vi "test_next_steps_json.vi"(8 "error in (no error)":errorcluster) -> (0 "error out":errorcluster)   [LabVIEW 2023, in "Easy.SequenceManager.Test.lvlib"]
uses:
  Easy.SequenceManager.Test.lvlib
  src/SequenceManager/SequenceManager.lvclass
  <vilib>/addons/_JKI Toolkits/Caraya/classes/Assert/Assert Equal Value and Type_Variant.vi
  <vilib>/addons/_JKI Toolkits/Caraya/classes/Test/Test.lvclass
  <vilib>/addons/_JKI Toolkits/Caraya/classes/Assert/Assert.lvclass
panel:
  in  "SequenceManager in":refnum<class "SequenceManager.lvclass">
  # "Connector Pane"
  # "Locals"
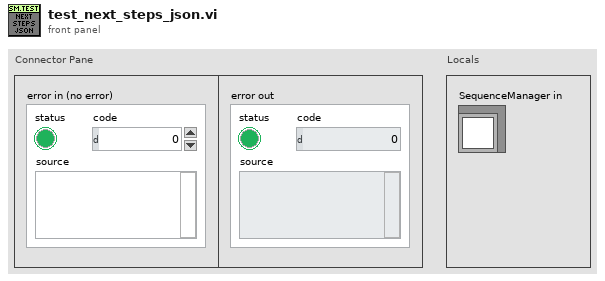
[diagram p1: front panel]
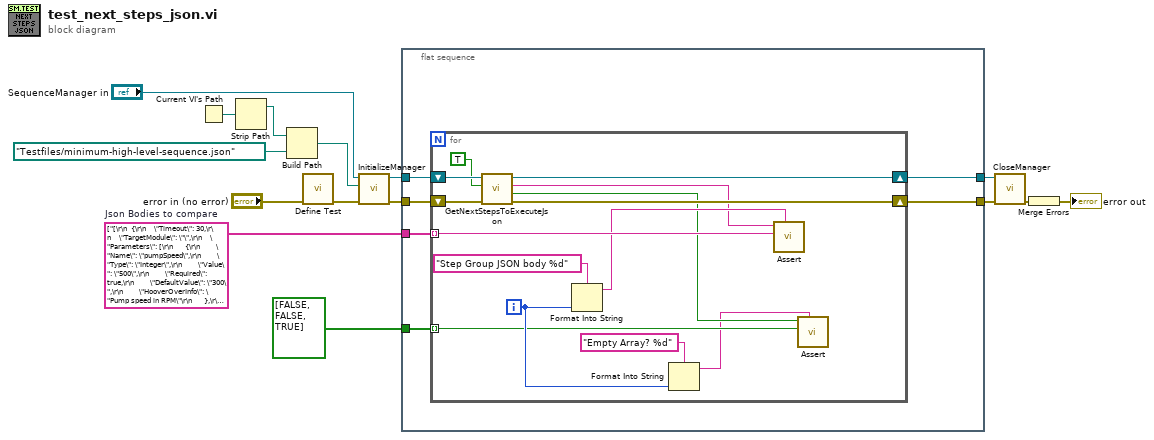
[diagram p0: block diagram]
diagram:
  w2 = string[] ["[\r\n  {\r\n    \"Timeout\": 30,\r\n    \"TargetModule\": \"\",\r\n    \"Parameters\": [\r\n      {\r\n        \"Name\": \"pumpSpeed\",\r\n        \"Type\": \"Integer\",\r\n        \"Value\": \"500\",\r\n        \"Required\": true,\r\n        \"DefaultValue\": \"300\",\r\n        \"HooverOverInfo\": \"Pump speed in RPM\"\r\n      },\r\n      {\r\n        \"Name\": \"pumpMode\",\r\n        \"Type\": \"String\",\r\n        \"Value\": \"Auto\",\r\n        \"Required\": false,\r\n        \"DefaultValue\": \"Manual\",\r\n        \"HooverOverInfo\": \"Pump operation mode\"\r\n      }\r\n    ],\r\n    \"IsSynchronous\": true,\r\n    \"IsParallel\": false,\r\n    \"Name\": \"Fill Box With Stuff\",\r\n    \"Documentation\": \"Any documentation needed\"\r\n  }\r\n]", "[\r\n  {\r\n    \"Timeout\": 45,\r\n    \"TargetModule\": \"\",\r\n    \"Parameters\": [\r\n      {\r\n        \"Name\": \"axisTargetPosition1\",\r\n        \"Type\": \"Float\",\r\n        \"Value\": \"10.5\",\r\n        \"Required\": true,\r\n        \"DefaultValue\": \"0.0\",\r\n        \"HooverOverInfo\": \"Target position for the axis movement\"\r\n      },\r\n      {\r\n        \"Name\": \"axisSpeed1\",\r\n        \"Type\": \"Float\",\r\n        \"Value\": \"10.5\",\r\n        \"Required\": true,\r\n        \"DefaultValue\": \"0.0\",\r\n        \"HooverOverInfo\": \"Target position for the axis movement\"\r\n      },\r\n      {\r\n        \"Name\": \"axisTargetPosition2\",\r\n        \"Type\": \"Float\",\r\n        \"Value\": \"10.5\",\r\n        \"Required\": true,\r\n        \"DefaultValue\": \"0.0\",\r\n        \"HooverOverInfo\": \"Target position for the axis movement\"\r\n      },\r\n      {\r\n        \"Name\": \"axisSpeed2\",\r\n        \"Type\": \"Float\",\r\n        \"Value\": \"10.5\",\r\n        \"Required\": true,\r\n        \"DefaultValue\": \"0.0\",\r\n        \"HooverOverInfo\": \"Target position for the axis movement\"\r\n      }\r\n    ],\r\n    \"IsSynchronous\": false,\r\n    \"IsParallel\": false,\r\n    \"Name\": \"Compression\",\r\n    \"Documentation\": \"Any documentation needed\"\r\n  }\r\n]", "[]"]  # Json Bodies to compare
  n1 = Current VI's Path() -> (path=w14:path)
  n2 = Strip Path(path=w14) -> (stripped path=w8:path)  [unwired: 1 out]
  n3 = Build Path(base path=w8, name or relative path=path "Testfiles/minimum-high-level-sequence.json") -> (appended path=w9:path)
  n4 = call <vilib>:"Define Test.vi"("error in (no error)"="error in (no error)") -> ("error out"=w7:errorcluster)  [unwired: 9 in, 1 out]
  n5 = call-dynamic "InitializeManager.vi"("error in (no error)"=w7, "Path to JSON sequence file"=w9, "SequenceManager in"="SequenceManager in") -> ("error out"=w6:errorcluster, "SequenceManager out"=w10:refnum<class "SequenceManager.lvclass">)  [unwired: 7 in]
  n6 = flat-sequence {
    tunnel: w10 -> [w20]
    tunnel: w6 -> [w21]
    tunnel: [w19] -> w4
    tunnel: [w18] -> w3
    tunnel: w2 -> [w17]
    tunnel: bool[] [FALSE, FALSE, TRUE] ("Array") -> [w16]
    frame #0 {
      n7 = for {
        tunnel: w17 -> [w30] mode=indexing
        shift-right: [w32] -> w18
        shift-left: w21 -> [w35]
        shift-right: [w33] -> w19
        shift-left: w20 -> [w34]
        tunnel: w16 -> [w24] mode=indexing
        i -> [w25]
        n8 = call-dynamic "GetNextStepsToExecuteJson.vi"("error in (no error)"=w35, "beautify JSON?"=TRUE, "SequenceManager in"=w34) -> ("error out"=w32:errorcluster, "Empty Array?"=w23:bool, "GetNextStepsToExecuteAsJson"=w27:string, "SequenceManager out"=w33:refnum<class "SequenceManager.lvclass">)  [unwired: 5 in]
        n9 = Format Into String(format string="Step Group JSON body %d", w25) -> (resulting string=w28:string)  [unwired: 2 in, 1 out]
        n10 = Format Into String(format string="Empty Array? %d", w25) -> (resulting string=w22:string)  [unwired: 2 in, 1 out]
        n11 = call-poly <vilib>:"Assert.vi"("Label"=w28, "Y"=w30, "X"=w27) -> ()  [unwired: 7 in, 2 out]
        n12 = call-poly <vilib>:"Assert.vi"("Label"=w22, "Y"=w24, "X"=w23) -> ()  [unwired: 7 in, 2 out]
      }
    }
  }
  n13 = call-dynamic "CloseManager.vi"("error in (no error)"=w3, "SequenceManager in"=w4) -> ("error out"=w5:errorcluster)  [unwired: 8 in, 1 out]
  n14 = Merge Errors(w5) -> (→"error out":errorcluster)
